vi "Graphing template.vi"() -> ()   [LabVIEW 2020]
panel:
  out "Waveform Chart":dbl(graph)
  out "read buffer":string
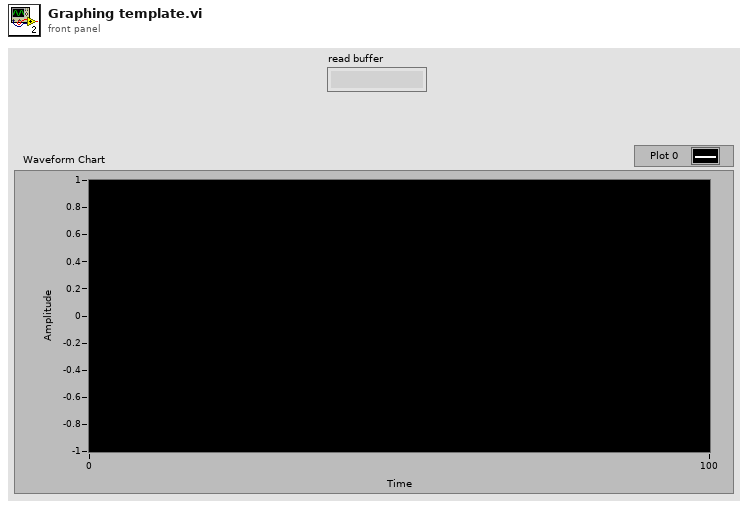
[diagram p1: front panel]
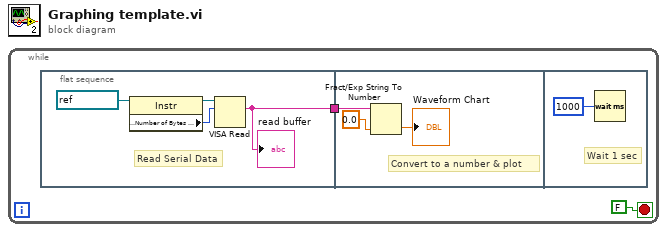
[diagram p0: block diagram]
diagram:
  n1 = while {
    stop <- FALSE stop-if-true
    n2 = flat-sequence {
      tunnel: [w3] -> w1
      tunnel: w1 -> [w9]
      frame #0 {
        # "Read Serial Data"
        n3 = property class="Instr"(reference=refnum<visa-resource-name> "COM4" ("VISA resource name")) -> (reference out=w5:refnum<visa-resource-name>, "Serial Settings:Number of Bytes at Serial Port"=w4:u32)  [unwired: 1 in, 1 out]
        n4 = VISA Read(VISA resource name=w5, byte count=w4) -> (read buffer=w3:string)  [unwired: 1 in, 3 out]
        "read buffer" <- w3
      }
      frame #1 {
        # "Convert to a number & plot"
        n5 = Fract/Exp String To Number(string=w9, default (0 dbl)=0.0 ("default (0 DBL)")) -> (number=→"Waveform Chart":dbl)  [unwired: 2 in, 1 out]
      }
      frame #2 {
        # "Wait 1 sec"
        n6 = Wait (ms)(milliseconds to wait=u32 1000) -> ()  [unwired: 1 out]
      }
    }
  }
